vi "_Adjust Calibration Table.vi"(1 "Calibration Table In":dbl[][](array[numeric]) format="%.2f", 2 "Adjustment Factor":dbl) -> (0 "Calibration Table Out":dbl[][](array[numeric]) format="%.2f")   [LabVIEW 2012]
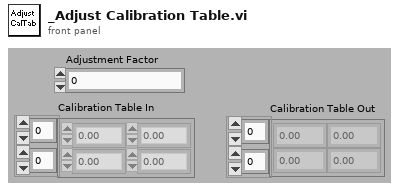
[diagram p1: front panel]
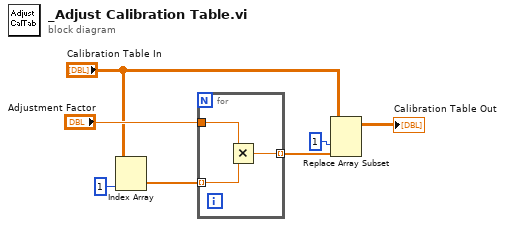
[diagram p0: block diagram]
diagram:
  n1 = Index Array(array="Calibration Table In", index (col)=1 ("disabled index (col)")) -> (element=w6:dbl[])  [unwired: 1 in]
  n2 = for {
    tunnel: w6 -> [w9] mode=indexing
    tunnel: "Adjustment Factor" -> [w10]
    tunnel: [w8] -> w2 mode=indexing
    n3 = Multiply(x=w10, y=w9) -> (x*y=w8:dbl)
  }
  n4 = Replace Array Subset(array="Calibration Table In", new element=w2, index (col)=1 ("disabled index (col)")) -> (→"Calibration Table Out":dbl[][])  [unwired: 1 in]
